vi "AH2500_read_visa.vi"(4 "error in (no error)":errorcluster caption="Fehler (Eingang, kein Fehler)", 7 "VISA-AH2500A-address":refnum<visa-resource-name>) -> (0 "error out":errorcluster caption="Fehler (Ausgang)", 1 "loss":dbl=nan format="%.8f", 2 "capacitance":dbl=nan format="%.8f", 3 "VISA-AH2500A-address dub":refnum<visa-resource-name>)   [LabVIEW 2019]
panel:
  out "Vexc":dbl=nan format="%.8f"
  out "out string":string
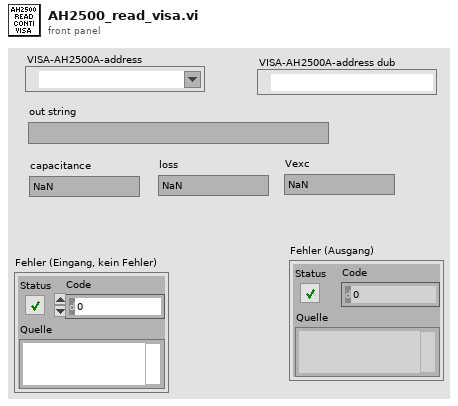
[diagram p1: front panel]
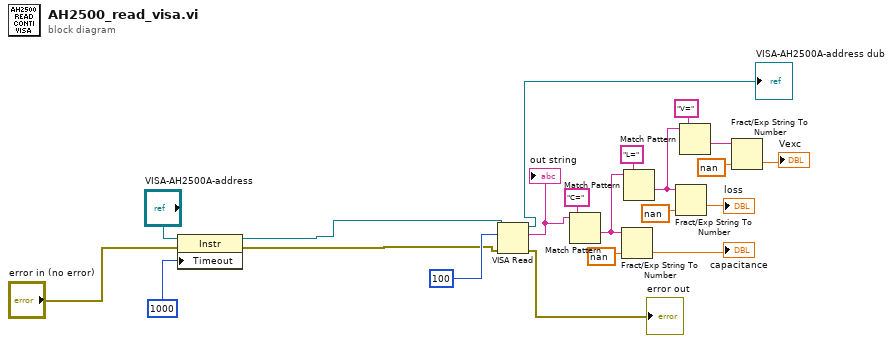
[diagram p0: block diagram]
diagram:
  n1 = property class="Instr"(reference="VISA-AH2500A-address", error in="error in (no error)", "Timeout"=u32 1000) -> (reference out=w3:refnum<visa-resource-name>, error out=w1:errorcluster)
  n2 = VISA Read(VISA resource name=w3, byte count=100, error in (no error)=w1) -> (VISA resource name out=→"VISA-AH2500A-address dub":refnum<visa-resource-name>, read buffer=w6:string, error out=→"error out":errorcluster)  [unwired: 1 out]
  "out string" <- w6
  n3 = Match Pattern(string=w6, regular expression="C=") -> (after substring=w16:string)  [unwired: 1 in, 3 out]
  n4 = Fract/Exp String To Number(string=w16, default (0 dbl)=nan) -> (number=→"capacitance":dbl)  [unwired: 2 in, 1 out]
  n5 = Match Pattern(string=w16, regular expression="L=") -> (after substring=w11:string)  [unwired: 1 in, 3 out]
  n6 = Fract/Exp String To Number(string=w11, default (0 dbl)=nan) -> (number=→"loss":dbl)  [unwired: 2 in, 1 out]
  n7 = Match Pattern(string=w11, regular expression="V=") -> (after substring=w14:string)  [unwired: 1 in, 3 out]
  n8 = Fract/Exp String To Number(string=w14, default (0 dbl)=nan) -> (number=→"Vexc":dbl)  [unwired: 2 in, 1 out]
